vi "AprilTagStandard52h13Codes.vi"() -> (0 "Codes":i64[](array[numeric])=[8987, 11941, 13418, 17849, 31142, 32619, -19624, -6331, -423, 5485, 14347, -3925, 3460, 18230, -29582, -20720, 2364, -27724, -23293, 18063, -7881, 22421, -8382, 7197, -5668, 29613, -21153, -10960, 1994, -20690] format="%.0x", 1 "Layout":string="xxxxdddxxxxxxdddddddxxxdbbbbbbbdxxdbwwwwwbdxddbwdddwbddddbwdddwbddddbwdddwbddxdbwwwwwbdxxdbbbbbbbdxxxdddddddxxxxxxdddxxxx")   [LabVIEW 2020, in "feature_detection.lvlib"]
uses:
  feature_detection.lvlib
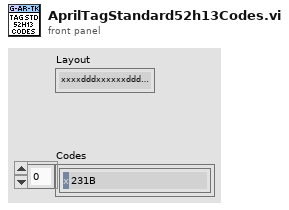
[diagram p1: front panel]
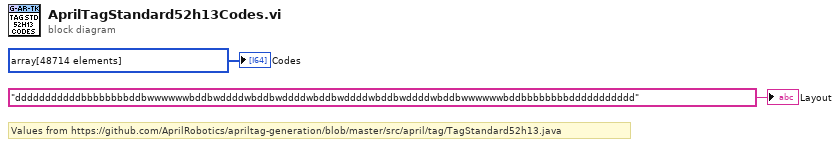
[diagram p0: block diagram]
diagram:
  # "Values from https://github.com/AprilRobotics/apriltag-generation/blob/master/src/april/tag/TagStandard52h13.java"
  "Codes" <- i64[] array[48714 elements] ("Array")
  "Layout" <- "dddddddddddbbbbbbbbddbwwwwwwbddbwddddwbddbwddddwbddbwddddwbddbwddddwbddbwwwwwwbddbbbbbbbbddddddddddd" ("String")
